vi "Hide Parent Holder.vi"(8 "Error In":errorcluster, 11 "Child Folder In":path=path "") -> (0 "Error Out":errorcluster, 3 "Child Folder Out":path)   [LabVIEW 2018, in "Tools Menu.lvlib"]
uses:
  Tools Menu.lvlib
  kernel32.dll
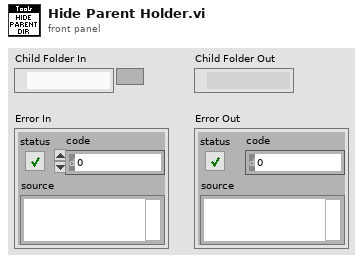
[diagram p1: front panel]
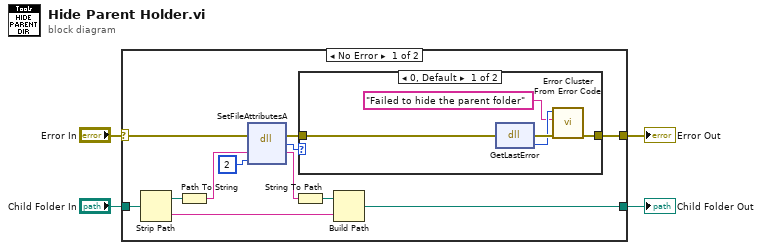
[diagram p0: block diagram]
diagram:
  n1 = case shown="No Error" "Error In" {
    selector: "Error In" -> [w8 w24]
    tunnel: [w16 w23] -> w4
    tunnel: "Child Folder In" -> [w11 w23]
    tunnel: [w5 w24] -> w2
    frame No Error {
      n2 = Strip Path(path=w11) -> (stripped path=w12:path, name=w15:string)
      n3 = Path To String(path=w12) -> (string=w13:string)
      n4 = dll-call lib="kernel32.dll" fn="SetFileAttributesA"(error in=w8, "lpFileName"=w13, "dwFileAttributes"=u32 2) -> (error out=w6:errorcluster, "return type"=w7:i32, "lpFileName"=w9:string)  [unwired: 3 in, 1 out]
      n5 = String To Path(string=w9) -> (path=w14:path)
      n6 = case shown="0, Default" w7 {
        tunnel: w6 -> [w20 w22]
        tunnel: [w21 w22] -> w5
        frame 0, Default {
          n7 = dll-call lib="kernel32.dll" fn="GetLastError"(error in=w20) -> (error out=w19:errorcluster, "return type"=w18:u32)  [unwired: 2 in, 1 out]
          n8 = call <vilib>:"Error Cluster From Error Code.vi"("error in (no error)"=w19, "error message (\"\")"="Failed to hide the parent folder" ("error message (\"\")"), "error code (0)"=w18) -> ("error out"=w21:errorcluster)  [unwired: 6 in]
        }
        frame 1 {
        }
      }
      n9 = Build Path(base path=w14, name or relative path=w15) -> (appended path=w16:path)
    }
    frame Error {
    }
  }
  "Child Folder Out" <- w4
  "Error Out" <- w2
